vi "Simple Filter Try 1.vi"(8 "error in":errorcluster) -> (0 "error out":errorcluster)   [LabVIEW 2014]
doc: "DEMO 423 - Digital Filter for Arduino\n\nSimple shows how to implement filter in diagram and after rewrite it into arduino code. This filter is also able to run on desktop application for testing."
uses:
  <vilib>/LabVIEW Universal Transcriptor/LabVIEW for Arduino Math Library/Arduino Math.lvlib
panel:
  out "signal in":sgl[](graph)
  in  "signal type":u16(ring) items=["sine", "user"]
  out "signal out":sgl[](graph)
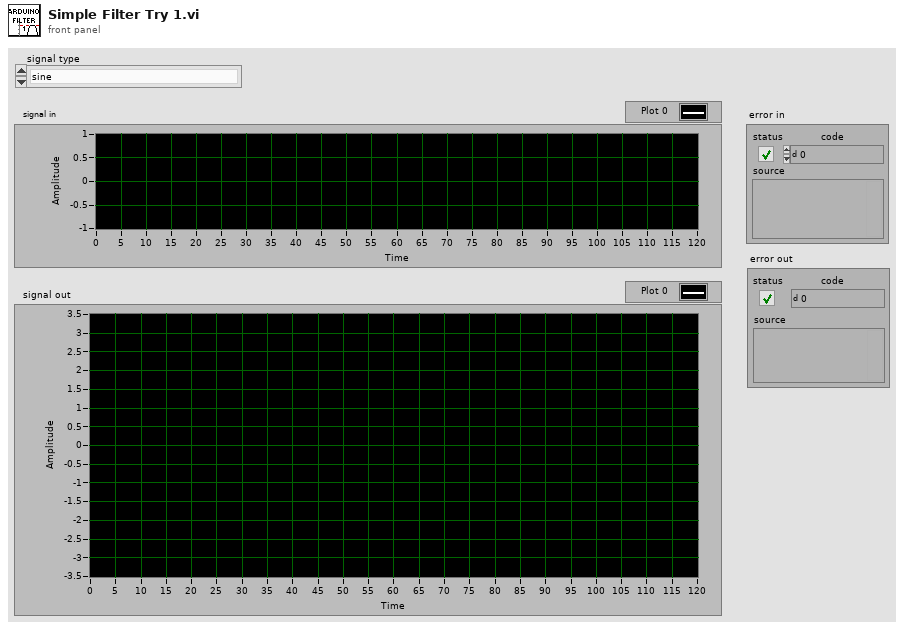
[diagram p1: front panel]
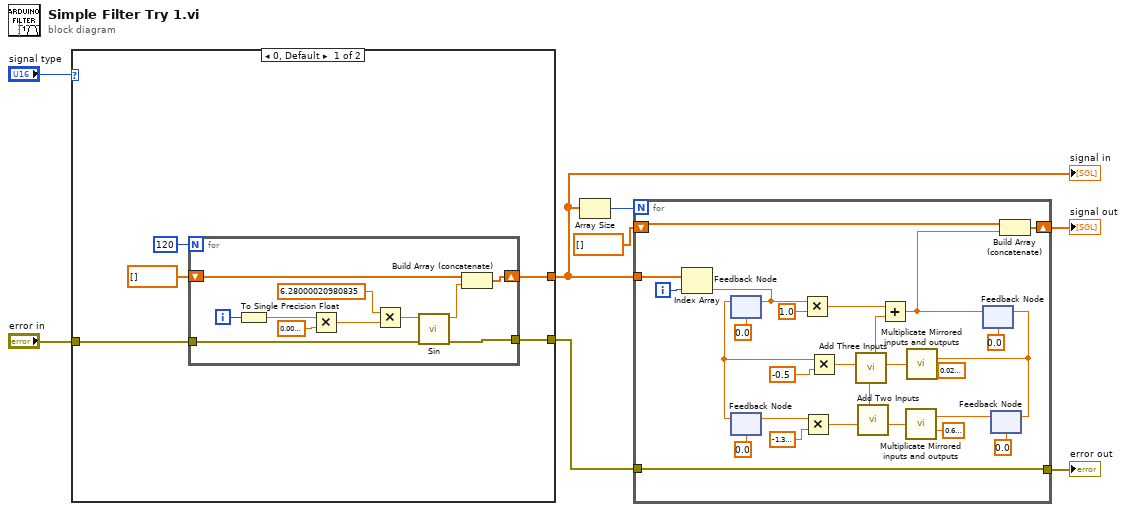
[diagram p0: block diagram]
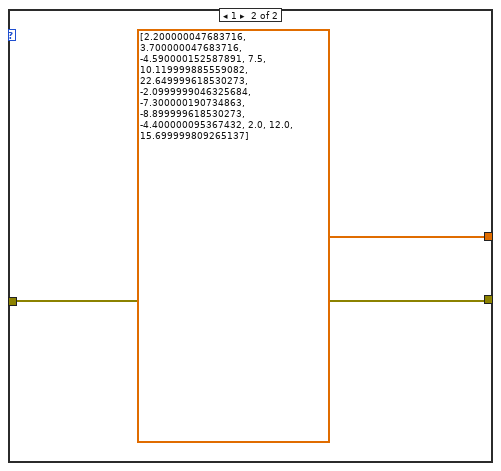
[diagram p2: hidden frame]
diagram:
  n1 = case shown="0, Default" "signal type" {
    tunnel: [w10 sgl[] [2.2, 3.7, -4.59, 7.5, 10.12, 22.65, -2.1, -7.3, -8.9, -4.4, 2.0, 12.0, 15.7]] -> w4
    tunnel: "error in" -> [w12 w25]
    tunnel: [w9 w25] -> w2
    frame 0, Default {
      n2 = for {
        N: 120 -> [_]
        tunnel: w12 -> [w24]
        shift-right: [w17] -> w10
        shift-left: sgl[] [] -> [w15]
        tunnel: [w14] -> w9
        i -> [w22]
        n3 = To Single Precision Float(number=w22) -> (single precision float=w20:sgl)
        n4 = Multiply(x=w20, y=sgl 0.01) -> (x*y=w19:sgl)
        n5 = Multiply(x=sgl 6.28, y=w19) -> (x*y=w18:sgl)
        n6 = call <vilib>:"Sin.vi"("Error In"=w24, "x"=w18) -> ("Error Out"=w14:errorcluster, "sin(x)"=w16:sgl)  [unwired: 8 in]
        n7 = Build Array (concatenate)(w15, w16) -> (w17:sgl[])
      }
    }
    frame 1 {
    }
  }
  "signal in" <- w4
  n8 = Array Size(array=w4) -> (size(s)=w8:i32)
  n9 = for {
    N: w8 -> [_]
    tunnel: w4 -> [w53]
    shift-right: [w51] -> w3
    shift-left: sgl[] [] -> [w50]
    tunnel: [w27] -> w1
    tunnel: w2 -> [w27]
    i -> [w52]
    n10 = Index Array(array=w53, index=w52) -> (element=w43:sgl)
    n11 = feedback #1(sgl 0.0 ("sin(x)")) -> (w38:sgl)
    n12 = feedback-in #1(w43) -> ()
    n13 = feedback #2(sgl 0.0 ("sin(x)")) -> (w35:sgl)
    n14 = feedback-in #2(w38) -> ()
    n15 = Multiply(x=w43, y=sgl 1.0) -> (x*y=w42:sgl)
    n16 = Multiply(x=w35, y=sgl -1.4) -> (x*y=w36:sgl)
    n17 = Multiply(x=w38, y=sgl -0.5) -> (x*y=w39:sgl)
    n18 = feedback #3(sgl 0.0 ("sin(x)")) -> (w32:sgl)
    n19 = call "Multiplicate Mirrored inputs and outputs.vi"("in 1"=w32, "in 2"=sgl 0.03) -> ("out"=w33:sgl)  [unwired: 13 in]
    n20 = feedback #4(sgl 0.0 ("sin(x)")) -> (w29:sgl)
    n21 = call "Multiplicate Mirrored inputs and outputs.vi"("in 1"=w29, "in 2"=sgl 0.7) -> ("out"=w28:sgl)  [unwired: 13 in]
    n22 = call "Add Two Inputs.vi"("in 2"=w28, "in 1"=w36) -> ("Numeric"=w44:sgl)  [unwired: 9 in]
    n23 = call "Add Three Inputs.vi"("in 2"=w33, "in 3"=w44, "in 1"=w39) -> ("Numeric"=w45:sgl)  [unwired: 8 in]
    n24 = Add(x=w42, y=w45) -> (x+y=w34:sgl)
    n25 = feedback-in #3(w34) -> ()
    n26 = feedback-in #4(w32) -> ()
    n27 = Build Array (concatenate)(w50, w34) -> (w51:sgl[])
  }
  "error out" <- w1
  "signal out" <- w3
